vi "Lab Panel V5.25.vi"() -> ()   [LabVIEW 2017] (continued)
              }
              frame #9 {
                n2523 = case shown="True" w4672 {
                  tunnel: w4676 -> [_ w4681]
                  tunnel: w4675 -> [_ w4680]
                  tunnel: w4674 -> [_ w4678]
                  tunnel: w4673 -> [_ w4677]
                  frame False {
                  }
                  frame True {
                    n2524 = local read "DISP LAB05-2"() -> (w4682:T4)
                    n2525 = local read "SIG LAB05-2"() -> (w4683:T2)
                    n2526 = local read "ON L05-2"() -> (w4679:cluster{"amps":dbl, "volts":dbl, "pf":dbl})
                    n2527 = Unbundle(w4683) -> ("AMPS"=w4689:dbl, "VOLTS"=w4687:dbl, "PF"=w4686:dbl, "Tmp Live"=w4685:dbl, "Tmp Neut"=w4688:dbl)
                    n2528 = Unbundle(w4682) -> ("CYCLE"=w4684:dbl)  [unwired: 2 out]
                    n2529 = stacked-sequence {
                      tunnel: w4689 -> [w4693 w4712]
                      tunnel: w4688 -> [_ w4711]
                      tunnel: w4687 -> [w4692 w4710]
                      tunnel: w4686 -> [w4691 w4709]
                      tunnel: w4685 -> [_ w4708]
                      tunnel: w4684 -> [_ w4707]
                      tunnel: w4681 -> [_ w4706]
                      tunnel: w4680 -> [w4694 _]
                      tunnel: w4679 -> [w4690 w4704]
                      tunnel: w4678 -> [_ w4705]
                      tunnel: w4677 -> [_ w4700]
                      frame #0 {
                        n2530 = case shown="True" w4694 {
                          tunnel: w4693 -> [_ w4699]
                          tunnel: w4692 -> [_ w4698]
                          tunnel: w4691 -> [_ w4697]
                          tunnel: w4690 -> [_ w4695]
                          frame False {
                          }
                          frame True {
                            n2531 = Bundle(cluster=w4695, "amps"=w4699, "volts"=w4698, "pf"=w4697) -> (w4696:cluster{"amps":dbl, "volts":dbl, "pf":dbl})
                            n2532 = local write "ON L05-2"(w4696) -> ()
                          }
                        }
                      }
                      frame #1 {
                        n2533 = Unbundle(w4704) -> ("amps"=w4703:dbl, "volts"=w4702:dbl, "pf"=w4701:dbl)
                        n2534 = case shown="True" w4705 {
                          tunnel: w4712 -> [_ w4744]
                          tunnel: w4711 -> [_ w4751]
                          tunnel: w4710 -> [_ _]
                          tunnel: w4709 -> [_ _]
                          tunnel: w4708 -> [_ w4750]
                          tunnel: w4707 -> [_ w4749]
                          tunnel: w4706 -> [_ w4714]
                          tunnel: w4703 -> [_ w4746]
                          tunnel: w4702 -> [_ w4745]
                          tunnel: w4701 -> [_ w4743]
                          tunnel: w4700 -> [_ w4735]
                          frame False {
                          }
                          frame True {
                            n2535 = local read "TDMS LAB05-2"() -> (w4748:refnum<k34>)
                            n2536 = Build Array(w4745) -> (w4740:dbl[])
                            n2537 = Build Array(w4743) -> (w4739:dbl[])
                            n2538 = Build Array(w4750) -> (w4738:dbl[])
                            n2539 = Build Array(w4751) -> (w4737:dbl[])
                            n2540 = Build Array(w4746) -> (w4742:dbl[])
                            n2541 = Build Array(w4744) -> (w4741:dbl[])
                            n2542 = Build Array(w4749) -> (w4736:dbl[])
                            n2543 = Build Array("AMPS ON", "AMPS OFF", "VOLTS", "PF", "TEMP Live", "TEMP Neut", "CYCLE") -> (w4719:string[])
                            n2544 = Bundle By Name("Y"=w4742, "t0"=w4735) -> (w4734:waveform(dbl))  [unwired: 1 in]
                            n2545 = Bundle By Name("Y"=w4741, "t0"=w4735) -> (w4733:waveform(dbl))  [unwired: 1 in]
                            n2546 = Bundle By Name("Y"=w4740, "t0"=w4735) -> (w4732:waveform(dbl))  [unwired: 1 in]
                            n2547 = Bundle By Name("Y"=w4739, "t0"=w4735) -> (w4731:waveform(dbl))  [unwired: 1 in]
                            n2548 = Bundle By Name("Y"=w4738, "t0"=w4735) -> (w4730:waveform(dbl))  [unwired: 1 in]
                            n2549 = Bundle By Name("Y"=w4737, "t0"=w4735) -> (w4729:waveform(dbl))  [unwired: 1 in]
                            n2550 = Bundle By Name("Y"=w4736, "t0"=w4735) -> (w4728:waveform(dbl))  [unwired: 1 in]
                            n2551 = Build Array(w4734, w4733, w4732, w4731, w4730, w4729, w4728) -> (w4727:waveform(dbl)[])
                            n2552 = TDMS Write(0:w4748, 5:"TEST VALUES", 7:w4719, 9:w4727) -> (4:w4718:refnum<k34>, 6:w4717:string, 15:w4716:errorcluster)  [unwired: 2 in, 1 out]
                            n2553 = TDMS Write(0:w4718, 5:w4717, 7:"TIME", 9:w4714, 11:w4716) -> (15:w4713:errorcluster)  [unwired: 1 in, 3 out]
                            n2554 = local write "data file error"(w4713) -> ()
                          }
                        }
                      }
                    }
                  }
                }
              }
            }
          }
          frame #14 {
            # "display test values on chart"
            n2555 = local read "jig cycle"() -> (w4756:dbl)
            n2556 = local read "on loops"() -> (w4758:dbl)
            n2557 = Add(x=w4758, y=2) -> (x+y=w4755:dbl)
            n2558 = Equal?(x=w4756, y=1) -> (x = y?=w4754:bool)
            n2559 = Equal?(x=w4756, y=w4755) -> (x = y?=w4753:bool)
            n2560 = Or(x=w4754, y=w4753) -> (x .or. y?=w4752:bool)
            "graph flag" <- w4752
            n2561 = global write "Global display 3.vi" "graph flag"(w4752) -> ()
            n2562 = case shown="True" w4752 {
              frame False {
              }
              frame True {
                n2563 = local read "SIG LAB05-1"() -> (w4801:T2)
                n2564 = local read "SIG LAB04-2"() -> (w4802:T2)
                n2565 = local read "SIG LAB05-2"() -> (w4800:T2)
                n2566 = local read "SIG LAB04-1"() -> (w4803:T2)
                n2567 = local read "SIG LAB03-1"() -> (w4805:T2)
                n2568 = local read "SIG LAB03-2"() -> (w4804:T2)
                n2569 = local read "SIG LAB01-1"() -> (w4809:T2)
                n2570 = local read "SIG LAB02-2"() -> (w4806:T2)
                n2571 = local read "SIG LAB02-1"() -> (w4807:T2)
                n2572 = local read "SIG LAB01-2"() -> (w4808:T2)
                n2573 = Unbundle(w4802) -> ("AMPS"=w4792:dbl, "VOLTS"=w4782:dbl, "Tmp Live"=w4772:dbl, "Tmp Neut"=w4762:dbl)  [unwired: 1 out]
                n2574 = Unbundle(w4801) -> ("AMPS"=w4791:dbl, "VOLTS"=w4781:dbl, "Tmp Live"=w4771:dbl, "Tmp Neut"=w4761:dbl)  [unwired: 1 out]
                n2575 = Unbundle(w4800) -> ("AMPS"=w4790:dbl, "VOLTS"=w4780:dbl, "Tmp Live"=w4770:dbl, "Tmp Neut"=w4760:dbl)  [unwired: 1 out]
                n2576 = Unbundle(w4803) -> ("AMPS"=w4793:dbl, "VOLTS"=w4783:dbl, "Tmp Live"=w4773:dbl, "Tmp Neut"=w4763:dbl)  [unwired: 1 out]
                n2577 = Unbundle(w4804) -> ("AMPS"=w4794:dbl, "VOLTS"=w4784:dbl, "Tmp Live"=w4774:dbl, "Tmp Neut"=w4764:dbl)  [unwired: 1 out]
                n2578 = Unbundle(w4805) -> ("AMPS"=w4795:dbl, "VOLTS"=w4785:dbl, "Tmp Live"=w4775:dbl, "Tmp Neut"=w4765:dbl)  [unwired: 1 out]
                n2579 = Unbundle(w4806) -> ("AMPS"=w4796:dbl, "VOLTS"=w4786:dbl, "Tmp Live"=w4776:dbl, "Tmp Neut"=w4766:dbl)  [unwired: 1 out]
                n2580 = Unbundle(w4807) -> ("AMPS"=w4797:dbl, "VOLTS"=w4787:dbl, "Tmp Live"=w4777:dbl, "Tmp Neut"=w4767:dbl)  [unwired: 1 out]
                n2581 = Unbundle(w4809) -> ("AMPS"=w4799:dbl, "VOLTS"=w4789:dbl, "Tmp Live"=w4779:dbl, "Tmp Neut"=w4769:dbl)  [unwired: 1 out]
                n2582 = Unbundle(w4808) -> ("AMPS"=w4798:dbl, "VOLTS"=w4788:dbl, "Tmp Live"=w4778:dbl, "Tmp Neut"=w4768:dbl)  [unwired: 1 out]
                n2583 = stacked-sequence {
                  tunnel: w4799 -> [w4841 _ _]
                  tunnel: w4798 -> [w4840 _ _]
                  tunnel: w4797 -> [w4831 _ _]
                  tunnel: w4796 -> [w4830 _ _]
                  tunnel: w4795 -> [w4820 _ _]
                  tunnel: w4794 -> [w4819 _ _]
                  tunnel: w4793 -> [_ w4864 _]
                  tunnel: w4792 -> [_ w4863 _]
                  tunnel: w4791 -> [_ w4853 _]
                  tunnel: w4790 -> [_ w4852 _]
                  tunnel: w4789 -> [w4838 _ _]
                  tunnel: w4788 -> [w4837 _ _]
                  tunnel: w4787 -> [w4828 _ _]
                  tunnel: w4786 -> [w4827 _ _]
                  tunnel: w4785 -> [w4818 _ _]
                  tunnel: w4784 -> [w4817 _ _]
                  tunnel: w4783 -> [_ w4862 _]
                  tunnel: w4782 -> [_ w4861 _]
                  tunnel: w4781 -> [_ w4851 _]
                  tunnel: w4780 -> [_ w4850 _]
                  tunnel: w4779 -> [w4835 _ _]
                  tunnel: w4778 -> [w4833 _ _]
                  tunnel: w4777 -> [w4824 _ _]
                  tunnel: w4776 -> [w4822 _ _]
                  tunnel: w4775 -> [w4816 _ _]
                  tunnel: w4774 -> [w4814 _ _]
                  tunnel: w4773 -> [_ w4860 _]
                  tunnel: w4772 -> [_ w4858 _]
                  tunnel: w4771 -> [_ w4849 _]
                  tunnel: w4770 -> [_ w4847 _]
                  tunnel: w4769 -> [w4834 _ _]
                  tunnel: w4768 -> [w4832 _ _]
                  tunnel: w4767 -> [w4823 _ _]
                  tunnel: w4766 -> [w4821 _ _]
                  tunnel: w4765 -> [w4815 _ _]
                  tunnel: w4764 -> [w4813 _ _]
                  tunnel: w4763 -> [_ w4859 _]
                  tunnel: w4762 -> [_ w4857 _]
                  tunnel: w4761 -> [_ w4848 _]
                  tunnel: w4760 -> [_ w4846 _]
                  frame #0 {
                    n2584 = Merge Signals(w4841, w4840) -> (→"LAB01 AMPS":dynamicdata)
                    n2585 = Merge Signals(w4838, w4837) -> (→"LAB01 VOLTS":dynamicdata)
                    n2586 = Merge Signals(w4818, w4817) -> (→"LAB03 VOLTS":dynamicdata)
                    n2587 = Merge Signals(w4835, w4834, w4833, w4832) -> (→"LAB01 deg C":dynamicdata)
                    n2588 = Merge Signals(w4831, w4830) -> (→"LAB02 AMPS":dynamicdata)
                    n2589 = Merge Signals(w4824, w4823, w4822, w4821) -> (→"LAB02 deg C":dynamicdata)
                    n2590 = Merge Signals(w4816, w4815, w4814, w4813) -> (→"LAB03 deg C":dynamicdata)
                    n2591 = Merge Signals(w4828, w4827) -> (→"LAB02 VOLTS":dynamicdata)
                    n2592 = Merge Signals(w4820, w4819) -> (→"LAB03 AMPS":dynamicdata)
                  }
                  frame #1 {
                    n2593 = Merge Signals(w4851, w4850) -> (→"LAB05 VOLTS":dynamicdata)
                    n2594 = Merge Signals(w4864, w4863) -> (→"LAB04 AMPS":dynamicdata)
                    n2595 = Merge Signals(w4853, w4852) -> (→"LAB05 AMPS":dynamicdata)
                    n2596 = Merge Signals(w4849, w4848, w4847, w4846) -> (→"LAB05 deg C":dynamicdata)
                    n2597 = Merge Signals(w4860, w4859, w4858, w4857) -> (→"LAB04 deg C":dynamicdata)
                    n2598 = Merge Signals(w4862, w4861) -> (→"LAB04 VOLTS":dynamicdata)
                  }
                  frame #2 {
                    n2599 = local read "LAB05 VOLTS"() -> (w4872:dynamicdata)
                    n2600 = local read "LAB04 VOLTS"() -> (w4873:dynamicdata)
                    n2601 = local read "LAB05 AMPS"() -> (w4878:dynamicdata)
                    n2602 = local read "LAB02 VOLTS"() -> (w4875:dynamicdata)
                    n2603 = local read "LAB03 VOLTS"() -> (w4874:dynamicdata)
                    n2604 = local read "LAB01 VOLTS"() -> (w4876:dynamicdata)
                    n2605 = local read "LAB04 AMPS"() -> (w4879:dynamicdata)
                    n2606 = local read "LAB03 AMPS"() -> (w4880:dynamicdata)
                    n2607 = local read "LAB03 deg C"() -> (w4868:dynamicdata)
                    n2608 = local read "LAB02 AMPS"() -> (w4881:dynamicdata)
                    n2609 = local read "LAB04 deg C"() -> (w4867:dynamicdata)
                    n2610 = local read "LAB05 deg C"() -> (w4866:dynamicdata)
                    n2611 = local read "LAB02 deg C"() -> (w4869:dynamicdata)
                    n2612 = local read "LAB01 deg C"() -> (w4870:dynamicdata)
                    n2613 = local read "LAB01 AMPS"() -> (w4882:dynamicdata)
                    n2614 = Merge Signals(w4870, w4869, w4868, w4867, w4866) -> (w4865:dynamicdata)
                    n2615 = Merge Signals(w4882, w4881, w4880, w4879, w4878) -> (w4877:dynamicdata)
                    n2616 = Merge Signals(w4876, w4875, w4874, w4873, w4872) -> (w4871:dynamicdata)
                    n2617 = global write "Global display 3.vi" "graph volts"(w4871) -> ()
                    n2618 = global write "Global display 3.vi" "graph deg C"(w4865) -> ()
                    n2619 = global write "Global display 3.vi" "graph amps"(w4877) -> ()
                  }
                }
              }
            }
          }
          frame #15 {
            # "check for amps fail"
            # "check for cycle test & temperature rise fail conditions"
            n2620 = local read "on loops"() -> (w4909:dbl)
            n2621 = local read "jig cycle"() -> (w4906:dbl)
            n2622 = local read "jig cycle"() -> (w4911:dbl)
            n2623 = Add(x=w4909, y=3.0) -> (x+y=w4907:dbl)
            n2624 = Equal?(x=w4906, y=w4907) -> (x = y?=w4902:bool)
            n2625 = local read "Fail Loops"() -> (w4883:dbl)
            n2626 = Equal?(x=w4911, y=1.0) -> (x = y?=w4904:bool)
            n2627 = global write "Global 1.vi" "fail count"(w4883) -> ()
            n2628 = stacked-sequence {
              tunnel: w4905 -> [w4914 _ _ _ _ _ _ _ _ _]
              tunnel: w4904 -> [w4915 w4935 w4955 w4975 w4995 w5015 w5035 w5055 w5075 w5095]
              tunnel: w4903 -> [w4912 _ _ _ _ _ _ _ _ _]
              tunnel: w4902 -> [w4913 w4934 w4954 w4974 w4994 w5014 w5034 w5054 w5074 w5094]
              tunnel: w4901 -> [_ w4933 _ _ _ _ _ _ _ _]
              tunnel: w4900 -> [_ w4932 _ _ _ _ _ _ _ _]
              tunnel: w4899 -> [_ _ w4953 _ _ _ _ _ _ _]
              tunnel: w4898 -> [_ _ w4952 _ _ _ _ _ _ _]
              tunnel: w4897 -> [_ _ _ w4973 _ _ _ _ _ _]
              tunnel: w4896 -> [_ _ _ w4972 _ _ _ _ _ _]
              tunnel: w4895 -> [_ _ _ _ w4993 _ _ _ _ _]
              tunnel: w4894 -> [_ _ _ _ w4992 _ _ _ _ _]
              tunnel: w4893 -> [_ _ _ _ _ w5013 _ _ _ _]
              tunnel: w4892 -> [_ _ _ _ _ w5012 _ _ _ _]
              tunnel: w4891 -> [_ _ _ _ _ _ w5033 _ _ _]
              tunnel: w4890 -> [_ _ _ _ _ _ w5032 _ _ _]
              tunnel: w4889 -> [_ _ _ _ _ _ _ w5053 _ _]
              tunnel: w4888 -> [_ _ _ _ _ _ _ w5052 _ _]
              tunnel: w4887 -> [_ _ _ _ _ _ _ _ w5073 _]
              tunnel: w4886 -> [_ _ _ _ _ _ _ _ w5072 _]
              tunnel: w4885 -> [_ _ _ _ _ _ _ _ _ w5093]
              tunnel: w4884 -> [_ _ _ _ _ _ _ _ _ w5092]
              frame #0 {
                # "LAB01-1"
                n2629 = case shown="True" w4912 {
                  tunnel: w4915 -> [_ w4928]
                  tunnel: w4914 -> [_ w4925]
                  tunnel: w4913 -> [_ w4924]
                  frame False {
                  }
                  frame True {
                    n2630 = local read "TEMP START LAB01-1"() -> (w4930:cluster{"TL":dbl, "TN":dbl})
                    n2631 = local read "RESULT LAB01-1"() -> (w4919:bool)
                    n2632 = local read "FAIL LAB01-1"() -> (w4922:cluster{"LO":dbl, "HI":dbl})
                    n2633 = local read "TDMS LAB01-1"() -> (w4929:refnum<k34>)
                    n2634 = local read "SET LAB01-1"() -> (w4926:T5)
                    n2635 = local read "DISP LAB01-1"() -> (w4927:T4)
                    n2636 = local read "SIG LAB01-1"() -> (w4931:T2)
                    n2637 = Bundle("FAIL LAB01-1"=w4922, "SIG LAB01-1"=w4931, "TEMP START LAB01-1"=w4930, "DISP LAB01-1"=w4927, "SET LAB01-1"=w4926, "TDMS LAB01-1"=w4929) -> (w4916:T33)  [unwired: 1 in]
                    n2638 = call "sub vi - cycle&temp fail v7.vi"("Amps Lo?"=w4928, "Input Cluster"=w4916, "SELECT"=w4925, "Amps Hi?"=w4924, "Result In"=w4919) -> ("(FAIL) out"=w4921:cluster{"FAIL LO":dbl, "FAIL HI":dbl}, "(DISP) out"=w4917:T4, "T-RISE"=w4918:cluster{"T-RISE (L)":dbl, "T-RISE (N)":dbl}, "Result Out"=w4920:bool, "file error"=w4923:errorcluster)  [unwired: 10 in]
                    n2639 = local write "TEMP RISE LAB01-1"(w4918) -> ()
                    n2640 = local write "FAIL LAB01-1"(w4921) -> ()
                    n2641 = local write "DISP LAB01-1"(w4917) -> ()
                    n2642 = local write "RESULT LAB01-1"(w4920) -> ()
                    n2643 = local write "data file error"(w4923) -> ()
                  }
                }
              }
              frame #1 {
                # "LAB01-2"
                n2644 = case shown="True" w4933 {
                  tunnel: w4935 -> [_ w4948]
                  tunnel: w4932 -> [_ w4945]
                  tunnel: w4934 -> [_ w4944]
                  frame False {
                  }
                  frame True {
                    n2645 = local read "TEMP START LAB01-2"() -> (w4950:cluster{"TL":dbl, "TN":dbl})
                    n2646 = local read "FAIL LAB01-2"() -> (w4941:cluster{"LO":dbl, "HI":dbl})
                    n2647 = local read "TDMS LAB01-2"() -> (w4949:refnum<k34>)
                    n2648 = local read "SET LAB01-2"() -> (w4946:T5)
                    n2649 = local read "DISP LAB01-2"() -> (w4947:T4)
                    n2650 = local read "RESULT LAB01-2"() -> (w4938:bool)
                    n2651 = local read "SIG LAB01-2"() -> (w4951:T2)
                    n2652 = Bundle("FAIL LAB01-2"=w4941, "SIG LAB01-2"=w4951, "TEMP START LAB01-2"=w4950, "DISP LAB01-2"=w4947, "SET LAB01-2"=w4946, "TDMS LAB01-2"=w4949) -> (w4936:T34)  [unwired: 1 in]
                    n2653 = call "sub vi - cycle&temp fail v7.vi"("Amps Lo?"=w4948, "Input Cluster"=w4936, "SELECT"=w4945, "Amps Hi?"=w4944, "Result In"=w4938) -> ("(FAIL) out"=w4940:cluster{"FAIL LO":dbl, "FAIL HI":dbl}, "(DISP) out"=w4943:T4, "T-RISE"=w4937:cluster{"T-RISE (L)":dbl, "T-RISE (N)":dbl}, "Result Out"=w4939:bool, "file error"=w4942:errorcluster)  [unwired: 10 in]
                    n2654 = local write "TEMP RISE LAB01-2"(w4937) -> ()
                    n2655 = local write "FAIL LAB01-2"(w4940) -> ()
                    n2656 = local write "DISP LAB01-2"(w4943) -> ()
                    n2657 = local write "RESULT LAB01-2"(w4939) -> ()
                    n2658 = local write "data file error"(w4942) -> ()
                  }
                }
              }
              frame #2 {
                # "LAB02-1"
                n2659 = case shown="True" w4953 {
                  tunnel: w4955 -> [_ w4968]
                  tunnel: w4952 -> [_ w4965]
                  tunnel: w4954 -> [_ w4964]
                  frame False {
                  }
                  frame True {
                    n2660 = local read "TEMP START LAB02-1"() -> (w4970:cluster{"TL":dbl, "TN":dbl})
                    n2661 = local read "FAIL LAB02-1"() -> (w4961:cluster{"LO":dbl, "HI":dbl})
                    n2662 = local read "TDMS LAB02-1"() -> (w4969:refnum<k34>)
                    n2663 = local read "SET LAB02-1"() -> (w4966:T5)
                    n2664 = local read "DISP LAB02-1"() -> (w4967:T4)
                    n2665 = local read "SIG LAB02-1"() -> (w4971:T2)
                    n2666 = local read "RESULT LAB02-1"() -> (w4958:bool)
                    n2667 = Bundle("FAIL LAB02-1"=w4961, "SIG LAB02-1"=w4971, "TEMP START LAB02-1"=w4970, "DISP LAB02-1"=w4967, "SET LAB02-1"=w4966, "TDMS LAB02-1"=w4969) -> (w4956:T35)  [unwired: 1 in]
                    n2668 = call "sub vi - cycle&temp fail v7.vi"("Amps Lo?"=w4968, "Input Cluster"=w4956, "SELECT"=w4965, "Amps Hi?"=w4964, "Result In"=w4958) -> ("(FAIL) out"=w4960:cluster{"FAIL LO":dbl, "FAIL HI":dbl}, "(DISP) out"=w4963:T4, "T-RISE"=w4957:cluster{"T-RISE (L)":dbl, "T-RISE (N)":dbl}, "Result Out"=w4959:bool, "file error"=w4962:errorcluster)  [unwired: 10 in]
                    n2669 = local write "TEMP RISE LAB02-1"(w4957) -> ()
                    n2670 = local write "FAIL LAB02-1"(w4960) -> ()
                    n2671 = local write "DISP LAB02-1"(w4963) -> ()
                    n2672 = local write "RESULT LAB02-1"(w4959) -> ()
                    n2673 = local write "data file error"(w4962) -> ()
                  }
                }
              }
              frame #3 {
                # "LAB02-2"
                n2674 = case shown="True" w4973 {
                  tunnel: w4975 -> [_ w4988]
                  tunnel: w4972 -> [_ w4985]
                  tunnel: w4974 -> [_ w4984]
                  frame False {
                  }
                  frame True {
                    n2675 = local read "TEMP START LAB02-2"() -> (w4990:cluster{"TL":dbl, "TN":dbl})
                    n2676 = local read "FAIL LAB02-2"() -> (w4981:cluster{"LO":dbl, "HI":dbl})
                    n2677 = local read "TDMS LAB02-2"() -> (w4989:refnum<k34>)
                    n2678 = local read "SET LAB02-2"() -> (w4986:T5)
                    n2679 = local read "DISP LAB02-2"() -> (w4987:T4)
                    n2680 = local read "SIG LAB02-2"() -> (w4991:T2)
                    n2681 = local read "RESULT LAB02-2"() -> (w4978:bool)
                    n2682 = Bundle("FAIL LAB02-2"=w4981, "SIG LAB02-2"=w4991, "TEMP START LAB02-2"=w4990, "DISP LAB02-2"=w4987, "SET LAB02-2"=w4986, "TDMS LAB02-2"=w4989) -> (w4976:T36)  [unwired: 1 in]
                    n2683 = call "sub vi - cycle&temp fail v7.vi"("Amps Lo?"=w4988, "Input Cluster"=w4976, "SELECT"=w4985, "Amps Hi?"=w4984, "Result In"=w4978) -> ("(FAIL) out"=w4980:cluster{"FAIL LO":dbl, "FAIL HI":dbl}, "(DISP) out"=w4983:T4, "T-RISE"=w4977:cluster{"T-RISE (L)":dbl, "T-RISE (N)":dbl}, "Result Out"=w4979:bool, "file error"=w4982:errorcluster)  [unwired: 10 in]
                    n2684 = local write "TEMP RISE LAB02-2"(w4977) -> ()
                    n2685 = local write "FAIL LAB02-2"(w4980) -> ()
                    n2686 = local write "DISP LAB02-2"(w4983) -> ()
                    n2687 = local write "RESULT LAB02-2"(w4979) -> ()
                    n2688 = local write "data file error"(w4982) -> ()
                  }
                }
              }
              frame #4 {
                # "LAB03-1"
                n2689 = case shown="True" w4993 {
                  tunnel: w4995 -> [_ w5008]
                  tunnel: w4992 -> [_ w5005]
                  tunnel: w4994 -> [_ w5004]
                  frame False {
                  }
                  frame True {
                    n2690 = local read "TEMP START LAB03-1"() -> (w5010:cluster{"TL":dbl, "TN":dbl})
                    n2691 = local read "FAIL LAB03-1"() -> (w5001:cluster{"LO":dbl, "HI":dbl})
                    n2692 = local read "TDMS LAB03-1"() -> (w5009:refnum<k34>)
                    n2693 = local read "SET LAB03-1"() -> (w5006:T5)
                    n2694 = local read "DISP LAB03-1"() -> (w5007:T4)
                    n2695 = local read "SIG LAB03-1"() -> (w5011:T2)
                    n2696 = local read "RESULT LAB03-1"() -> (w4998:bool)
                    n2697 = Bundle("FAIL LAB03-1"=w5001, "SIG LAB03-1"=w5011, "TEMP START LAB03-1"=w5010, "DISP LAB03-1"=w5007, "SET LAB03-1"=w5006, "TDMS LAB03-1"=w5009) -> (w4996:T37)  [unwired: 1 in]
                    n2698 = call "sub vi - cycle&temp fail v7.vi"("Amps Lo?"=w5008, "Input Cluster"=w4996, "SELECT"=w5005, "Amps Hi?"=w5004, "Result In"=w4998) -> ("(FAIL) out"=w5000:cluster{"FAIL LO":dbl, "FAIL HI":dbl}, "(DISP) out"=w5003:T4, "T-RISE"=w4997:cluster{"T-RISE (L)":dbl, "T-RISE (N)":dbl}, "Result Out"=w4999:bool, "file error"=w5002:errorcluster)  [unwired: 10 in]
                    n2699 = local write "TEMP RISE LAB03-1"(w4997) -> ()
                    n2700 = local write "FAIL LAB03-1"(w5000) -> ()
                    n2701 = local write "DISP LAB03-1"(w5003) -> ()
                    n2702 = local write "RESULT LAB03-1"(w4999) -> ()
                    n2703 = local write "data file error"(w5002) -> ()
                  }
                }
              }
              frame #5 {
                # "LAB03-2"
                n2704 = case shown="True" w5013 {
                  tunnel: w5015 -> [_ w5028]
                  tunnel: w5012 -> [_ w5025]
                  tunnel: w5014 -> [_ w5024]
                  frame False {
                  }
                  frame True {
                    n2705 = local read "TEMP START LAB03-2"() -> (w5030:cluster{"TL":dbl, "TN":dbl})
                    n2706 = local read "FAIL LAB03-2"() -> (w5021:cluster{"LO":dbl, "HI":dbl})
                    n2707 = local read "TDMS LAB03-2"() -> (w5029:refnum<k34>)
                    n2708 = local read "SET LAB03-2"() -> (w5026:T5)
                    n2709 = local read "DISP LAB03-2"() -> (w5027:T4)
                    n2710 = local read "RESULT LAB03-2"() -> (w5018:bool)
                    n2711 = local read "SIG LAB03-2"() -> (w5031:T2)
                    n2712 = Bundle("FAIL LAB03-2"=w5021, "SIG LAB03-2"=w5031, "TEMP START LAB03-2"=w5030, "DISP LAB03-2"=w5027, "SET LAB03-2"=w5026, "TDMS LAB03-2"=w5029) -> (w5016:T38)  [unwired: 1 in]
                    n2713 = call "sub vi - cycle&temp fail v7.vi"("Amps Lo?"=w5028, "Input Cluster"=w5016, "SELECT"=w5025, "Amps Hi?"=w5024, "Result In"=w5018) -> ("(FAIL) out"=w5020:cluster{"FAIL LO":dbl, "FAIL HI":dbl}, "(DISP) out"=w5023:T4, "T-RISE"=w5017:cluster{"T-RISE (L)":dbl, "T-RISE (N)":dbl}, "Result Out"=w5019:bool, "file error"=w5022:errorcluster)  [unwired: 10 in]
                    n2714 = local write "FAIL LAB03-2"(w5020) -> ()
                    n2715 = local write "TEMP RISE LAB03-2"(w5017) -> ()
                    n2716 = local write "DISP LAB03-2"(w5023) -> ()
                    n2717 = local write "RESULT LAB03-2"(w5019) -> ()
                    n2718 = local write "data file error"(w5022) -> ()
                  }
                }
              }
              frame #6 {
                # "LAB04-1"
                n2719 = case shown="True" w5033 {
                  tunnel: w5035 -> [_ w5048]
                  tunnel: w5032 -> [_ w5045]
                  tunnel: w5034 -> [_ w5044]
                  frame False {
                  }
                  frame True {
                    n2720 = local read "TEMP START LAB04-1"() -> (w5050:cluster{"TL":dbl, "TN":dbl})
                    n2721 = local read "FAIL LAB04-1"() -> (w5041:cluster{"LO":dbl, "HI":dbl})
                    n2722 = local read "TDMS LAB04-1"() -> (w5049:refnum<k34>)
                    n2723 = local read "SET LAB04-1"() -> (w5046:T5)
                    n2724 = local read "DISP LAB04-1"() -> (w5047:T4)
                    n2725 = local read "SIG LAB04-1"() -> (w5051:T2)
                    n2726 = local read "RESULT LAB04-1"() -> (w5038:bool)
                    n2727 = Bundle("FAIL LAB04-1"=w5041, "SIG LAB04-1"=w5051, "TEMP START LAB04-1"=w5050, "DISP LAB04-1"=w5047, "SET LAB04-1"=w5046, "TDMS LAB04-1"=w5049) -> (w5036:T39)  [unwired: 1 in]
                    n2728 = call "sub vi - cycle&temp fail v7.vi"("Amps Lo?"=w5048, "Input Cluster"=w5036, "SELECT"=w5045, "Amps Hi?"=w5044, "Result In"=w5038) -> ("(FAIL) out"=w5040:cluster{"FAIL LO":dbl, "FAIL HI":dbl}, "(DISP) out"=w5043:T4, "T-RISE"=w5037:cluster{"T-RISE (L)":dbl, "T-RISE (N)":dbl}, "Result Out"=w5039:bool, "file error"=w5042:errorcluster)  [unwired: 10 in]
                    n2729 = local write "TEMP RISE LAB04-1"(w5037) -> ()
                    n2730 = local write "FAIL LAB04-1"(w5040) -> ()
                    n2731 = local write "DISP LAB04-1"(w5043) -> ()
                    n2732 = local write "RESULT LAB04-1"(w5039) -> ()
                    n2733 = local write "data file error"(w5042) -> ()
                  }
                }
              }
              frame #7 {
                # "LAB04-2"
                n2734 = case shown="True" w5053 {
                  tunnel: w5055 -> [_ w5068]
                  tunnel: w5052 -> [_ w5065]
                  tunnel: w5054 -> [_ w5064]
                  frame False {
                  }
                  frame True {
                    n2735 = local read "TEMP START LAB04-2"() -> (w5070:cluster{"TL":dbl, "TN":dbl})
                    n2736 = local read "FAIL LAB04-2"() -> (w5061:cluster{"LO":dbl, "HI":dbl})
                    n2737 = local read "TDMS LAB04-2"() -> (w5069:refnum<k34>)
                    n2738 = local read "SET LAB04-2"() -> (w5066:T5)
                    n2739 = local read "DISP LAB04-2"() -> (w5067:T4)
                    n2740 = local read "SIG LAB04-2"() -> (w5071:T2)
                    n2741 = local read "RESULT LAB04-2"() -> (w5058:bool)
                    n2742 = Bundle("FAIL LAB04-2"=w5061, "SIG LAB04-2"=w5071, "TEMP START LAB04-2"=w5070, "DISP LAB04-2"=w5067, "SET LAB04-2"=w5066, "TDMS LAB04-2"=w5069) -> (w5056:T40)  [unwired: 1 in]
                    n2743 = call "sub vi - cycle&temp fail v7.vi"("Amps Lo?"=w5068, "Input Cluster"=w5056, "SELECT"=w5065, "Amps Hi?"=w5064, "Result In"=w5058) -> ("(FAIL) out"=w5060:cluster{"FAIL LO":dbl, "FAIL HI":dbl}, "(DISP) out"=w5063:T4, "T-RISE"=w5057:cluster{"T-RISE (L)":dbl, "T-RISE (N)":dbl}, "Result Out"=w5059:bool, "file error"=w5062:errorcluster)  [unwired: 10 in]
                    n2744 = local write "TEMP RISE LAB04-2"(w5057) -> ()
                    n2745 = local write "FAIL LAB04-2"(w5060) -> ()
                    n2746 = local write "DISP LAB04-2"(w5063) -> ()
                    n2747 = local write "RESULT LAB04-2"(w5059) -> ()
                    n2748 = local write "data file error"(w5062) -> ()
                  }
                }
              }
              frame #8 {
                # "LAB05-1"
                n2749 = case shown="True" w5073 {
                  tunnel: w5075 -> [_ w5088]
                  tunnel: w5072 -> [_ w5085]
                  tunnel: w5074 -> [_ w5084]
                  frame False {
                  }
                  frame True {
                    n2750 = local read "TEMP START LAB05-1"() -> (w5090:cluster{"TL":dbl, "TN":dbl})
                    n2751 = local read "FAIL LAB05-1"() -> (w5081:cluster{"LO":dbl, "HI":dbl})
                    n2752 = local read "TDMS LAB05-1"() -> (w5089:refnum<k34>)
                    n2753 = local read "SET LAB05-1"() -> (w5086:T5)
                    n2754 = local read "DISP LAB05-1"() -> (w5087:T4)
                    n2755 = local read "SIG LAB05-1"() -> (w5091:T2)
                    n2756 = local read "RESULT LAB05-1"() -> (w5078:bool)
                    n2757 = Bundle("FAIL LAB05-1"=w5081, "SIG LAB05-1"=w5091, "TEMP START LAB05-1"=w5090, "DISP LAB05-1"=w5087, "SET LAB05-1"=w5086, "TDMS LAB05-1"=w5089) -> (w5076:T41)  [unwired: 1 in]
                    n2758 = call "sub vi - cycle&temp fail v7.vi"("Amps Lo?"=w5088, "Input Cluster"=w5076, "SELECT"=w5085, "Amps Hi?"=w5084, "Result In"=w5078) -> ("(FAIL) out"=w5080:cluster{"FAIL LO":dbl, "FAIL HI":dbl}, "(DISP) out"=w5083:T4, "T-RISE"=w5077:cluster{"T-RISE (L)":dbl, "T-RISE (N)":dbl}, "Result Out"=w5079:bool, "file error"=w5082:errorcluster)  [unwired: 10 in]
                    n2759 = local write "TEMP RISE LAB05-1"(w5077) -> ()
                    n2760 = local write "FAIL LAB05-1"(w5080) -> ()
                    n2761 = local write "DISP LAB05-1"(w5083) -> ()
                    n2762 = local write "RESULT LAB05-1"(w5079) -> ()
                    n2763 = local write "data file error"(w5082) -> ()
                  }
                }
              }
              frame #9 {
                # "LAB05-2"
                n2764 = case shown="True" w5093 {
                  tunnel: w5095 -> [_ w5108]
                  tunnel: w5092 -> [_ w5105]
                  tunnel: w5094 -> [_ w5104]
                  frame False {
                  }
                  frame True {
                    n2765 = local read "TEMP START LAB05-2"() -> (w5110:cluster{"TL":dbl, "TN":dbl})
                    n2766 = local read "FAIL LAB05-2"() -> (w5101:cluster{"LO":dbl, "HI":dbl})
                    n2767 = local read "TDMS LAB05-2"() -> (w5109:refnum<k34>)
                    n2768 = local read "SET LAB05-2"() -> (w5106:T5)
                    n2769 = local read "DISP LAB05-2"() -> (w5107:T4)
                    n2770 = local read "SIG LAB05-2"() -> (w5111:T2)
                    n2771 = local read "RESULT LAB05-2"() -> (w5098:bool)
                    n2772 = Bundle("FAIL LAB05-2"=w5101, "SIG LAB05-2"=w5111, "TEMP START LAB05-2"=w5110, "DISP LAB05-2"=w5107, "SET LAB05-2"=w5106, "TDMS LAB05-2"=w5109) -> (w5096:T42)  [unwired: 1 in]
                    n2773 = call "sub vi - cycle&temp fail v7.vi"("Amps Lo?"=w5108, "Input Cluster"=w5096, "SELECT"=w5105, "Amps Hi?"=w5104, "Result In"=w5098) -> ("(FAIL) out"=w5100:cluster{"FAIL LO":dbl, "FAIL HI":dbl}, "(DISP) out"=w5103:T4, "T-RISE"=w5097:cluster{"T-RISE (L)":dbl, "T-RISE (N)":dbl}, "Result Out"=w5099:bool, "file error"=w5102:errorcluster)  [unwired: 10 in]
                    n2774 = local write "TEMP RISE LAB05-2"(w5097) -> ()
                    n2775 = local write "FAIL LAB05-2"(w5100) -> ()
                    n2776 = local write "DISP LAB05-2"(w5103) -> ()
                    n2777 = local write "RESULT LAB05-2"(w5099) -> ()
                    n2778 = local write "data file error"(w5102) -> ()
                  }
                }
              }
            }
          }
          frame #16 {
            # "run calibration routine"
            n2779 = local read "SET (cal)"() -> (w5112:bool)
            n2780 = case shown="True" w5112 {
              frame False {
              }
              frame True {
                n2781 = stacked-sequence {
                  seq-local: [w5113 _ _] -> [_ w5115 _]
                  frame #0 {
                    n2782 = call "CALIBRATION PASSWORD"() -> ("PASSWORD"=w5113:string)  [unwired: 17 in, 2 out]
                  }
                  frame #1 {
                    n2783 = Equal?(x=w5115, y="7777") -> (x = y?=w5114:bool)
                    n2784 = case shown="True" w5114 {
                      frame False {
                      }
                      frame True {
                        n2785 = stacked-sequence {
                          frame #0 {
                            n2786 = local read "Temp Test Cal"() -> (w5117:dbl)
                            n2787 = call "sub vi - calibration v2.vi"("Temp Test Cal"=w5117) -> ()  [unwired: 11 in]
                          }
                          frame #1 {
                            n2788 = call "sub vi - get calibration values v1.vi"() -> ("TEMP REF CAL"=w5118:dbl, "LAB01 (CAL)"=w5123:T14, "LAB02 (CAL)"=w5122:T15, "LAB03 (CAL)"=w5121:T14, "LAB04 (CAL)"=w5120:T14, "calibration file error out"=w5124:errorcluster, "LAB05 (CAL)"=w5119:T14)  [unwired: 9 in]
                            n2789 = local write "TEMP REF cal"(w5118) -> ()
                            n2790 = local write "cal file error out"(w5124) -> ()
                            n2791 = local write "CAL LAB04"(w5120) -> ()
                            n2792 = local write "CAL LAB05"(w5119) -> ()
                            n2793 = local write "CAL LAB01"(w5123) -> ()
                            n2794 = local write "CAL LAB02"(w5122) -> ()
                            n2795 = local write "CAL LAB03"(w5121) -> ()
                          }
                        }
                      }
                    }
                  }
                  frame #2 {
                    n2796 = local write "SET (cal)"(FALSE) -> ()
                  }
                }
              }
            }
          }
          frame #17 {
            # "save certain settings to file"
            n2797 = String To Path(string="c:\\crabtree\\Set Up\\") -> (path=w5127:path)
            n2798 = Build Path(base path=w5127, name or relative path="settings.bin") -> (appended path=w5129:path)
            n2799 = Build Path(base path=w5127, name or relative path="mail.bin") -> (appended path=w5126:path)
            n2800 = Create Folder(path (use dialog)=w5127) -> (error out=w5132:errorcluster)  [unwired: 2 in, 2 out]
            n2801 = call <vilib>:"Clear Errors.vi"("error in (no error)"=w5132) -> ()  [unwired: 5 in, 2 out]
            n2802 = stacked-sequence {
              seq-local: [w5144 _] -> [_ w5157]
              tunnel: w5129 -> [_ w5158]
              tunnel: w5126 -> [_ w5156]
              frame #0 {
                n2803 = local read "C drive data root dir"() -> (w5143:path)
                n2804 = local read "Select COM port"() -> (w5140:refnum<visa-resource-name>)
                n2805 = local read "Network Directory"() -> (w5149:path)
                n2806 = local read "SET LAB05-2"() -> (w5148:T5)
                n2807 = local read "SET LAB05-1"() -> (w5147:T5)
                n2808 = local read "SET LAB04-2"() -> (w5146:T5)
                n2809 = local read "SET LAB03-2"() -> (w5150:T5)
                n2810 = local read "SET LAB04-1"() -> (w5145:T5)
                n2811 = local read "SET LAB03-1"() -> (w5151:T5)
                n2812 = local read "SET LAB02-2"() -> (w5152:T5)
                n2813 = local read "SET LAB02-1"() -> (w5153:T5)
                n2814 = local read "Temp Delay Lps"() -> (w5139:dbl)
                n2815 = local read "Amps Fail level"() -> (w5135:dbl)
                n2816 = local read "SET LAB01-2"() -> (w5154:T5)
                n2817 = local read "Temp Test Cal"() -> (w5136:dbl)
                n2818 = local read "SET LAB01-1"() -> (w5155:T5)
                n2819 = local read "Temp Value"() -> (w5138:dbl)
                n2820 = local read "Mail Test File To:"() -> (w5134:string)
                n2821 = local read "Fail Loops"() -> (w5137:dbl)
                n2822 = local read "Mail Test Fail"() -> (w5133:bool)
                n2823 = local read "RATE (Hz)"() -> (w5142:dbl)
                n2824 = local read "SAMPLES"() -> (w5141:dbl)
                n2825 = Bundle("SET LAB01-1"=w5155, "SET LAB01-2"=w5154, "SET LAB02-1"=w5153, "SET LAB02-2"=w5152, "SET LAB03-1"=w5151, "SET LAB03-2"=w5150, "SET LAB04-1"=w5145, "SET LAB04-2"=w5146, "SET LAB05-1"=w5147, "SET LAB05-2"=w5148, "Network Directory"=w5149, "C drive data root dir"=w5143, "RATE (Hz)"=w5142, "SAMPLES"=w5141, "Select COM port"=w5140, "Temp Delay Lps"=w5139, "Temp Value"=w5138, "Fail Loops"=w5137, "Temp Test Cal"=w5136, "Amps Fail level"=w5135, "Mail Test File To:"=w5134, "Mail Test Fail"=w5133) -> (w5144:T22)  [unwired: 1 in]
              }
              frame #1 {
                n2826 = event shown="[1] \"SET LAB01-1\", \"SET LAB01-2\", \"SET LAB02-1\", \"SET LAB02-2\", \"SET LAB03-1\", \"SET LAB03-2\", \"SET LAB04-1\", \"SET LAB04-2\", \"SET LAB05-1\", \"SET LAB05-2\", \"Network Directory\", \"C drive data root dir\", \"RATE (Hz)\", \"SAMPLES\", \"Select COM port\", \"Temp Delay Lps\", \"Temp Value\", \"Fail Loops\", \"Temp Test Cal\", \"Amps Fail level\", \"Mail Test File To:\", \"Mail Test Fail\": Value Change" {
                  selector: _ -> [_ _ _]
                  dyn-events: _ -> [_ _ _]
                  timeout: 10.0 -> [_ _ _]
                  tunnel: w5158 -> [_ w5160 _]
                  tunnel: w5157 -> [_ w5161 _]
                  tunnel: w5156 -> [_ _ w5172]
                  event Timeout {
                    n2827 = event-data() -> ()  [unwired: 1 in, 3 out]
                  }
                  event "SET LAB01-1", "SET LAB01-2", "SET LAB02-1", "SET LAB02-2", "SET LAB03-1", "SET LAB03-2", "SET LAB04-1", "SET LAB04-2", "SET LAB05-1", "SET LAB05-2", "Network Directory", "C drive data root dir", "RATE (Hz)", "SAMPLES", "Select COM port", "Temp Delay Lps", "Temp Value", "Fail Loops", "Temp Test Cal", "Amps Fail level", "Mail Test File To:", "Mail Test Fail": Value Change {
                    n2828 = event-data() -> ()  [unwired: 1 in, 6 out]
                    n2829 = Open/Create/Replace File(file path (use dialog)=w5160, operation (0:open)=T17."replace or create") -> (refnum out=w5166:refnum<file>, error out=w5165:errorcluster)  [unwired: 4 in, 1 out]
                    n2830 = Write to Binary File(file (use dialog)=w5166, data=w5161, error in=w5165) -> (refnum out=w5164:refnum<file>, error out=w5163:errorcluster)  [unwired: 3 in, 1 out]
                    n2831 = Close File(refnum=w5164, error in=w5163) -> (error out=w5162:errorcluster)  [unwired: 1 out]
                    n2832 = local write "data file error"(w5162) -> ()
                  }
                  event "MAIL SETTINGS.OUT SERVER ADDRESS", "MAIL SETTINGS.FROM ACCOUNT", "MAIL SETTINGS.USER NAME", "MAIL SETTINGS.PASSWORD", "Auto Mail Send", "TO (string):": Value Change {
                    n2833 = event-data() -> ()  [unwired: 1 in, 6 out]
                    n2834 = local read "Auto Mail Send"() -> (w5169:bool)
                    n2835 = local read "MAIL SETTINGS"() -> (w5171:T7)
                    n2836 = local read "TO (string):"() -> (w5168:string)
                    n2837 = Open/Create/Replace File(file path (use dialog)=w5172, operation (0:open)=T17."replace or create") -> (refnum out=w5177:refnum<file>, error out=w5176:errorcluster)  [unwired: 4 in, 1 out]
                    n2838 = Bundle("MAIL SETTINGS"=w5171, "Auto Mail Send"=w5169, "TO (string):"=w5168) -> (w5170:T43)  [unwired: 1 in]
                    n2839 = Write to Binary File(file (use dialog)=w5177, data=w5170, error in=w5176) -> (refnum out=w5175:refnum<file>, error out=w5174:errorcluster)  [unwired: 3 in, 1 out]
                    n2840 = Close File(refnum=w5175, error in=w5174) -> (error out=w5173:errorcluster)  [unwired: 1 out]
                    n2841 = local write "data file error"(w5173) -> ()
                  }
                }
              }
            }
          }
          frame #18 {
            # "mail control"
            n2842 = local read "MAIL SETTINGS"() -> (w5194:T7)
            n2843 = local read "Auto Mail Send"() -> (w5180:bool)
            n2844 = Unbundle(w5194) -> ("OUT SERVER ADDRESS"=w5193:string, "FROM ACCOUNT"=w5192:string, "TEST MAIL"=w5191:bool)  [unwired: 4 out]
            n2845 = stacked-sequence {
              tunnel: "TO (string):" -> [_ w5233]
              tunnel: w5194 -> [w5199 w5232]
              tunnel: w5193 -> [w5198 w5231]
              tunnel: w5192 -> [w5197 w5230]
              tunnel: w5191 -> [w5196 _]
              tunnel: w5180 -> [_ w5229]
              tunnel: w5190 -> [_ w5228]
              tunnel: w5189 -> [_ w5227]
              tunnel: w5188 -> [_ w5226]
              tunnel: w5187 -> [_ w5225]
              tunnel: w5186 -> [_ w5224]
              tunnel: w5185 -> [_ w5223]
              tunnel: w5184 -> [_ w5222]
              tunnel: w5183 -> [_ w5221]
              tunnel: w5182 -> [_ w5220]
              tunnel: w5181 -> [_ w5219]
              tunnel: "TO (string):" -> [w5195 _]
              frame #0 {
                # "mail test"
                n2846 = case shown="True" w5196 {
                  tunnel: w5199 -> [_ w5203]
                  tunnel: w5195 -> [_ w5202]
                  tunnel: w5198 -> [_ w5201]
                  tunnel: w5197 -> [_ w5200]
                  frame False {
                  }
                  frame True {
                    n2847 = stacked-sequence {
                      seq-local: [_ _ w5213 _] -> [_ _ _ w5214]
                      tunnel: w5203 -> [w5206 _ _ w5218]
                      tunnel: w5202 -> [_ _ w5211 _]
                      tunnel: w5201 -> [_ _ w5209 _]
                      tunnel: w5200 -> [_ _ w5210 _]
                      frame #0 {
                        n2848 = Bundle(cluster=w5206, "TEST MAIL STATUS"="TEST START") -> (w5204:T7)  [unwired: 6 in]
                        n2849 = local write "MAIL SETTINGS"(w5204) -> ()
                      }
                      frame #1 {
                        n2850 = Wait (ms)(milliseconds to wait=500) -> ()  [unwired: 1 out]
                      }
                      frame #2 {
                        n2851 = call "Lab Send Mail Test.vi"("TO:"=w5211, "subject"="MAIL TEST FROM LAB PANEL", "from"=w5210, "out going server"=w5209, "message"="TEST MESSAGE") -> ("error out"=w5213:errorcluster)  [unwired: 10 in]
                      }
                      frame #3 {
                        n2852 = Bundle(cluster=w5218, "TEST MAIL"=FALSE, "TEST MAIL STATUS"="TEST END", "mail error"=w5214) -> (w5216:T7)  [unwired: 4 in]
                        n2853 = local write "MAIL SETTINGS"(w5216) -> ()
                      }
                    }
                  }
                }
              }
              frame #1 {
                # "mail report"
                n2854 = stacked-sequence {
                  seq-local: [_ w5276 _ _] -> [_ _ _ w5466]
                  seq-local: [_ _ w5379 _] -> [_ _ _ w5456]
                  seq-local: [w5243 _ _ _] -> [_ w5293 _ _]
                  seq-local: [w5242 _ _ _] -> [_ w5292 _ _]
                  seq-local: [w5240 _ _ _] -> [_ w5290 _ _]
                  seq-local: [w5241 _ _ _] -> [_ w5291 _ _]
                  seq-local: [w5239 _ _ _] -> [_ w5289 _ _]
                  seq-local: [w5238 _ _ _] -> [_ w5284 _ _]
                  seq-local: [w5237 _ _ _] -> [_ w5285 _ _]
                  seq-local: [w5236 _ _ _] -> [_ w5286 _ _]
                  seq-local: [w5235 _ _ _] -> [_ w5287 _ _]
                  seq-local: [w5234 _ _ _] -> [_ w5288 _ _]
                  tunnel: w5233 -> [_ _ _ w5467]
                  tunnel: w5232 -> [_ _ _ w5450]
                  tunnel: w5231 -> [_ _ _ w5464]
                  tunnel: w5230 -> [_ _ _ w5463]
                  tunnel: w5229 -> [w5274 _ _ w5458]
                  tunnel: w5228 -> [_ _ w5409 _]
                  tunnel: w5227 -> [_ _ w5406 _]
                  tunnel: w5226 -> [_ _ w5405 _]
                  tunnel: w5225 -> [_ _ w5404 _]
                  tunnel: w5224 -> [_ _ w5403 _]
                  tunnel: w5223 -> [_ _ w5402 _]
                  tunnel: w5222 -> [_ _ w5401 _]
                  tunnel: w5221 -> [_ _ w5400 _]
                  tunnel: w5220 -> [_ _ w5399 _]
                  tunnel: w5219 -> [_ _ w5398 _]
                  frame #0 {
                    n2855 = case shown="False" w5274 {
                      frame False {
                        n2856 = local write "mail control"("") -> ()
                      }
                      frame True {
                      }
                    }
                    n2857 = local read "SET LAB01-1"() -> (w5273:T5)
                    n2858 = local read "SET LAB01-2"() -> (w5272:T5)
                    n2859 = local read "SET LAB02-1"() -> (w5271:T5)
                    n2860 = local read "SET LAB02-2"() -> (w5270:T5)
                    n2861 = local read "SET LAB03-1"() -> (w5269:T5)
                    n2862 = local read "SET LAB04-1"() -> (w5267:T5)
                    n2863 = local read "SET LAB05-1"() -> (w5265:T5)
                    n2864 = local read "SET LAB03-2"() -> (w5268:T5)
                    n2865 = local read "SET LAB04-2"() -> (w5266:T5)
                    n2866 = local read "SET LAB05-2"() -> (w5264:T5)
                    n2867 = Unbundle(w5269) -> ("DESCRIPTION"=w5249:string)  [unwired: 4 out]
                    n2868 = Unbundle(w5268) -> ("DESCRIPTION"=w5248:string)  [unwired: 4 out]
                    n2869 = Unbundle(w5267) -> ("DESCRIPTION"=w5247:string)  [unwired: 4 out]
                    n2870 = Unbundle(w5264) -> ("DESCRIPTION"=w5244:string)  [unwired: 4 out]
                    n2871 = Unbundle(w5270) -> ("DESCRIPTION"=w5250:string)  [unwired: 4 out]
                    n2872 = Unbundle(w5266) -> ("DESCRIPTION"=w5246:string)  [unwired: 4 out]
                    n2873 = Unbundle(w5273) -> ("DESCRIPTION"=w5262:string)  [unwired: 4 out]
                    n2874 = Unbundle(w5271) -> ("DESCRIPTION"=w5251:string)  [unwired: 4 out]
                    n2875 = Unbundle(w5265) -> ("DESCRIPTION"=w5245:string)  [unwired: 4 out]
                    n2876 = Unbundle(w5272) -> ("DESCRIPTION"=w5252:string)  [unwired: 4 out]
                    n2877 = Concatenate Strings("[LAB05-2/", w5244) -> (w5234:string)
                    n2878 = Concatenate Strings("[LAB05-1/", w5245) -> (w5235:string)
                    n2879 = Concatenate Strings("[LAB04-2/", w5246) -> (w5236:string)
                    n2880 = Concatenate Strings("[LAB03-2/", w5248) -> (w5238:string)
                    n2881 = Concatenate Strings("[LAB04-1/", w5247) -> (w5237:string)
                    n2882 = Concatenate Strings("[LAB03-1/", w5249) -> (w5239:string)
                    n2883 = Concatenate Strings("[LAB01-2/", w5252) -> (w5242:string)
                    n2884 = Concatenate Strings("[LAB02-2/", w5250) -> (w5240:string)
                    n2885 = Concatenate Strings("[LAB01-1/", w5262) -> (w5243:string)
                    n2886 = Concatenate Strings("[LAB02-1/", w5251) -> (w5241:string)
                  }
                  frame #1 {
                    w5297 = "/"
                    w5298 = 2.0
                    n2887 = local read "DISP LAB01-2"() -> (w5377:T4)
                    n2888 = local read "DISP LAB01-1"() -> (w5378:T4)
                    n2889 = local read "DISP LAB02-1"() -> (w5376:T4)
                    n2890 = local read "DISP LAB03-2"() -> (w5373:T4)
                    n2891 = local read "DISP LAB02-2"() -> (w5375:T4)
                    n2892 = local read "DISP LAB03-1"() -> (w5374:T4)
                    n2893 = local read "DISP LAB04-2"() -> (w5371:T4)
                    n2894 = local read "DISP LAB04-1"() -> (w5372:T4)
                    n2895 = local read "DISP LAB05-1"() -> (w5370:T4)
                    n2896 = local read "DISP LAB05-2"() -> (w5369:T4)
                    n2897 = Unbundle(w5377) -> ("CYCLE"=w5361:dbl, "MINS"=w5360:dbl, "STATUS"=w5357:string)
                    n2898 = Unbundle(w5378) -> ("CYCLE"=w5366:dbl, "MINS"=w5365:dbl, "STATUS"=w5362:string)
                    n2899 = Unbundle(w5376) -> ("CYCLE"=w5354:dbl, "MINS"=w5353:dbl, "STATUS"=w5352:string)
                    n2900 = Unbundle(w5373) -> ("CYCLE"=w5341:dbl, "MINS"=w5340:dbl, "STATUS"=w5337:string)
                    n2901 = Unbundle(w5374) -> ("CYCLE"=w5346:dbl, "MINS"=w5345:dbl, "STATUS"=w5342:string)
                    n2902 = Unbundle(w5375) -> ("CYCLE"=w5351:dbl, "MINS"=w5350:dbl, "STATUS"=w5347:string)
